vi "CRYCal Measurement Confidence.vi"(4 "Harmonic":dbl[](array[numeric]), 5 "z":dbl[](array[numeric]), 6 "Fs":dbl format="%.2f", 7 "x":dbl[](array[numeric]), 8 "Total Noise":dbl[](array[numeric]), 9 "Freq resp curves":dbl[][](array[numeric]), 10 "Method":u16, 11 "HT Option":bool[](array[boolean])) -> (3 "Harmonic Track Out":T1(array[cluster]))   [LabVIEW 2013]
uses:
  <vilib>/Analysis/NI_AALBase.lvlib
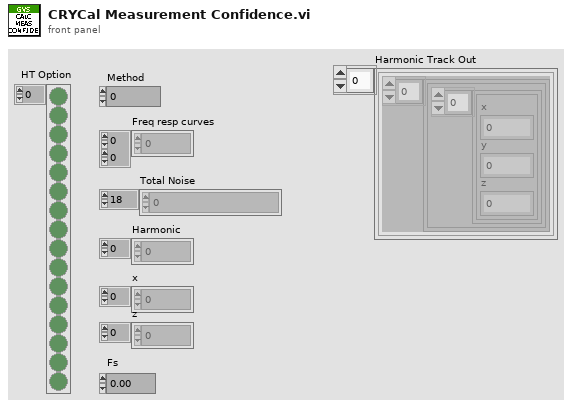
[diagram p1: front panel]
types:
  T1 = cluster{cluster{cluster{"x":dbl, "y":dbl, "z":dbl}[]}[]}[]
  T2 = cluster{"x":dbl, "standard deviation":dbl, "Z":dbl}[]
  T3 = cluster{cluster{"x":dbl, "standard deviation":dbl, "Z":dbl}[]}
  T4 = cluster{cluster{"x":dbl, "standard deviation":dbl, "Z":dbl}[]}[]
  T5 = cluster{"Freq resp curves clipped":cluster{cluster{"x":dbl, "y":dbl, "z":dbl}[]}[]}[]
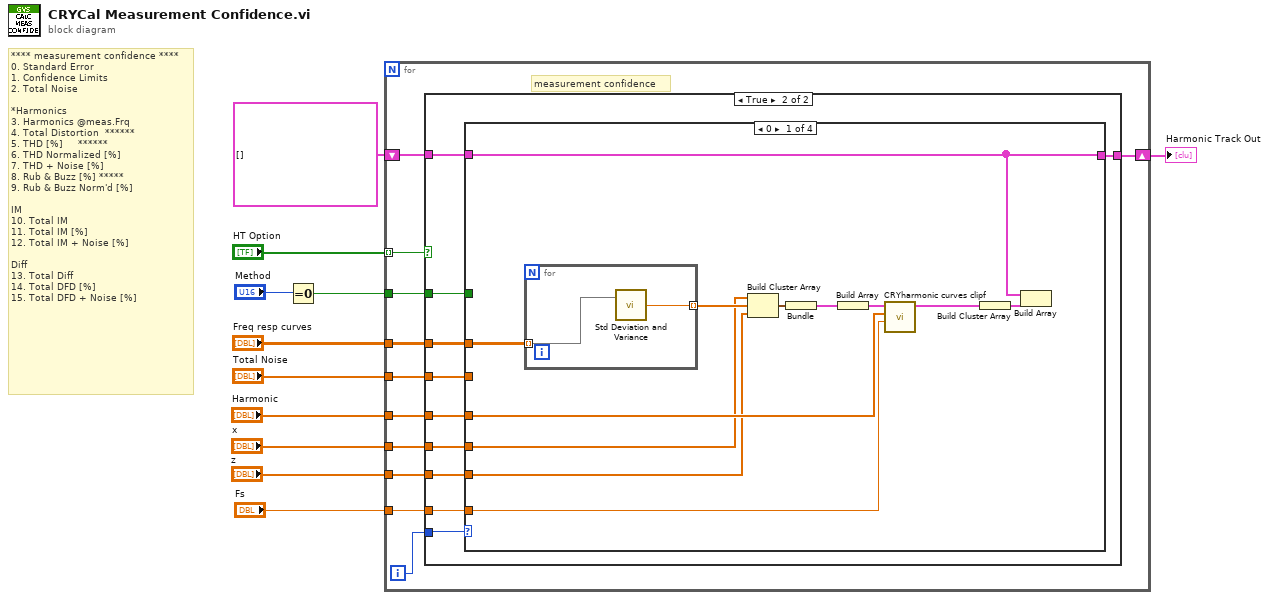
[diagram p0: block diagram]
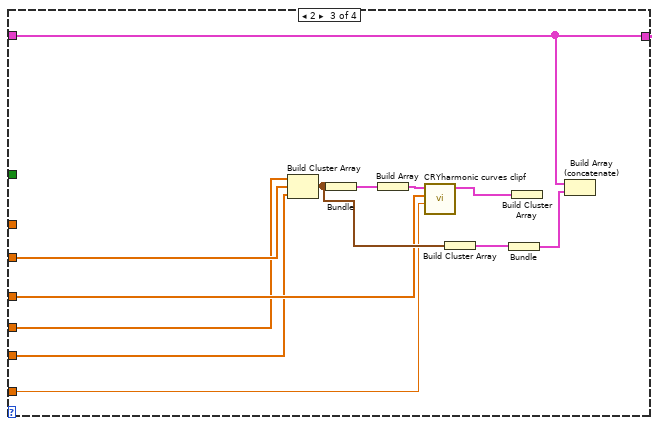
[diagram p4: hidden frame]
diagram:
  # "**** measurement confidence ****\n0. Standard Error\n1. Confidence Limits\n2. Total Noise\n\n*Harmonics\n3. Harmonics @meas.Frq\n4. Total Distortion  ******\n5. THD [%]     ******\n6. THD Normalized [%]\n7. THD + Noise [%]\n8. Rub & Buzz [%] *****\n9. Rub & Buzz Norm'd [%]\n\nIM\n10. Total IM\n11. Total IM [%]\n12. Total IM + Noise [%]\n\nDiff\n13. Total Diff\n14. Total DFD [%]\n15. Total DFD + Noise [%]"
  n1 = Equal To 0?(x="Method") -> (x = 0?=w10:bool)
  n2 = for {
    tunnel: "Freq resp curves" -> [w22]
    tunnel: w10 -> [w21]
    tunnel: "Total Noise" -> [w19]
    tunnel: "Harmonic" -> [w18]
    tunnel: "Fs" -> [w17]
    tunnel: "x" -> [w16]
    tunnel: "z" -> [w15]
    tunnel: "HT Option" -> [w12] mode=indexing
    shift-right: [w14] -> w2
    shift-left: cluster{cluster{cluster[]}[]}[] [] -> [w20]
    i -> [w13]
    # "measurement confidence"
    n3 = case shown="True" w12 {
      tunnel: w22 -> [_ w33]
      tunnel: w21 -> [_ w32]
      tunnel: w20 -> [w23 w31]
      tunnel: w19 -> [_ w30]
      tunnel: w18 -> [_ w29]
      tunnel: w17 -> [_ w28]
      tunnel: w16 -> [_ w27]
      tunnel: w15 -> [_ w26]
      tunnel: [w23 w25] -> w14
      tunnel: w13 -> [_ w24]
      frame False {
      }
      frame True {
        n4 = case shown="0" w24 {
          tunnel: w31 -> [w39 w48 w54 w61]
          tunnel: w33 -> [w45 _ _ _]
          tunnel: [w39 w48 w54 w61] -> w25
          tunnel: w32 -> [_ _ _ _]
          tunnel: w30 -> [_ _ w59 _]
          tunnel: w29 -> [w37 _ w52 _]
          tunnel: w28 -> [w36 _ w49 _]
          tunnel: w27 -> [w35 _ w51 _]
          tunnel: w26 -> [w34 _ w50 _]
          frame 0 {
            n5 = for {
              tunnel: w45 -> [w47] mode=indexing
              tunnel: [w46] -> w44 mode=indexing
              n6 = call <vilib>:"Std Deviation and Variance.vi"("X"=w47) -> ("standard deviation"=w46:dbl)  [unwired: 1 in, 2 out]
            }
            n7 = Build Cluster Array(w35, w44, w34) -> (w41:T2)
            n8 = Bundle(w41) -> (w42:T3)  [unwired: 1 in]
            n9 = Build Array(w42) -> (w43:T4)
            n10 = call "CRYharmonic curves clipf.vi"("Fs"=w36, "Harmonics"=w37, "Freq resp curves"=w43) -> ("Freq resp curves clipped"=w38:cluster{cluster{"x":dbl, "y":dbl, "z":dbl}[]}[])  [unwired: 8 out]
            n11 = Build Cluster Array(w38) -> (w40:T5)
            n12 = Build Array(w39, w40) -> ()  [unwired: 1 out]
          }
          frame 1 {
          }
          frame 2 {
            n13 = Build Cluster Array(w51, w59, w50) -> (w57:cluster{"x":dbl, dbl, "Z":dbl}[])
            n14 = Bundle(w57) -> (w58:cluster{cluster{"x":dbl, dbl, "Z":dbl}[]})  [unwired: 1 in]
            n15 = Build Array(w58) -> (w60:cluster{cluster{"x":dbl, dbl, "Z":dbl}[]}[])
            n16 = call "CRYharmonic curves clipf.vi"("Fs"=w49, "Harmonics"=w52, "Freq resp curves"=w60) -> ("Freq resp curves clipped"=w53:cluster{cluster{"x":dbl, "y":dbl, "z":dbl}[]}[])  [unwired: 8 out]
            n17 = Build Cluster Array(w57) -> (w56:cluster{cluster{"x":dbl, dbl, "Z":dbl}[]}[])
            n18 = Bundle(w56) -> (w55:cluster{cluster{cluster[]}[]})  [unwired: 1 in]
            n19 = Build Cluster Array(w53) -> ()  [unwired: 1 out]
            n20 = Build Array (concatenate)(w54, w55) -> ()  [unwired: 1 out]
          }
          frame Default {
          }
        }
      }
    }
  }
  "Harmonic Track Out" <- w2
